vi "Realtime Data (by ref).vi"(1 "New Data":dbl[][](array[numeric]), 2 "Enum":enum16{"Init", "Read", "Write"}(ring)) -> (0 "New Data":dbl[][](array[numeric]))   [LabVIEW 2023]
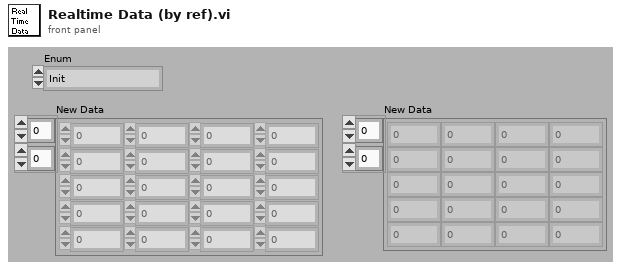
[diagram p1: front panel]
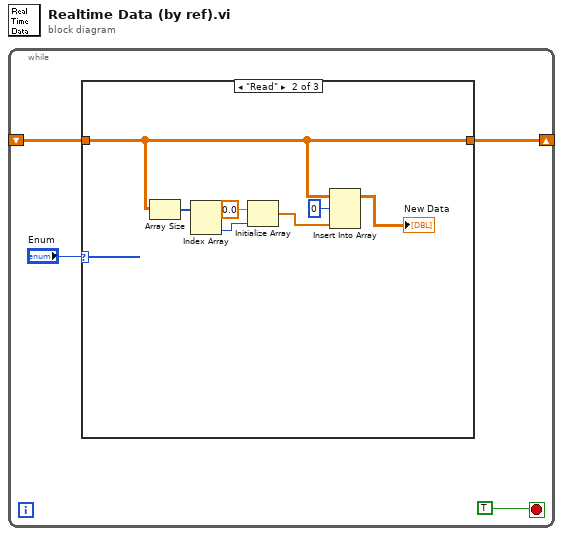
[diagram p0: block diagram]
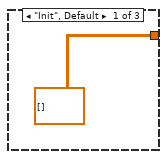
[diagram p2: hidden frame]
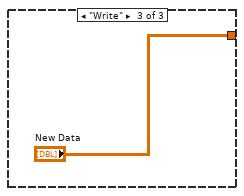
[diagram p3: hidden frame]
diagram:
  n1 = while {
    shift-right: [w2] -> _
    shift-left: _ -> [w1]
    stop <- TRUE ("stop") stop-if-true
    n2 = case shown="\"Read\"" "Enum" {
      tunnel: [dbl[][] [] w10 "New Data"] -> w2
      tunnel: w1 -> [_ w10 _]
      frame "Init", Default {
      }
      frame "Read" {
        n3 = Array Size(array=w10) -> (size(s)=w12:i32[])
        n4 = Index Array(array=w12) -> (element #2=w6:i32)  [unwired: 2 in, 1 out]
        n5 = Initialize Array(0.0 ("element"), w6) -> (w9:dbl[])
        n6 = Insert Into Array(array=w10, index (row)=0, new element=w9) -> (→"New Data":dbl[][])  [unwired: 1 in]
      }
      frame "Write" {
      }
    }
  }
